vi "ActionOnStart.vi"(8 "error in (no error)":errorcluster, 11 "Channel Manager in":refnum<class "Channel Manager.lvclass">) -> (0 "error out":errorcluster, 3 "Channel Manager out":refnum<class "Channel Manager.lvclass">)   [LabVIEW 2024, in "Embedded TDMS Logger Engine.lvlib" / "Channel Manager.lvclass"]
uses:
  Channel Manager.lvclass
  Channel Manager.lvclass/Channel Manager.ctl
  Shared/File Classes/File/File.lvclass
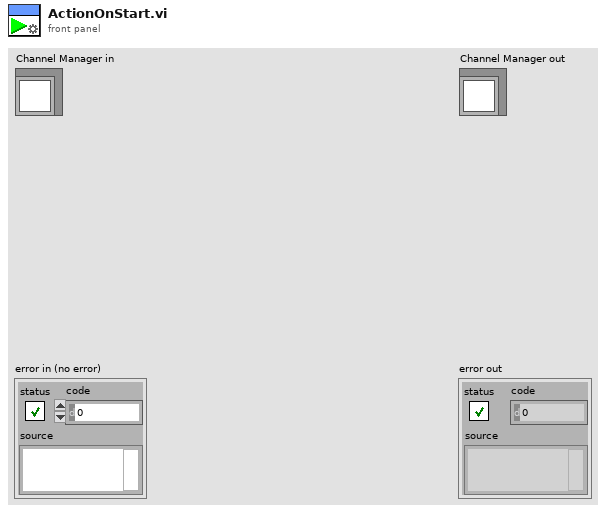
[diagram p1: front panel]
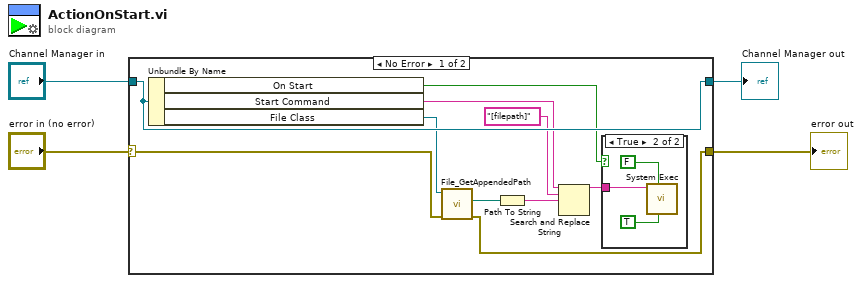
[diagram p0: block diagram]
diagram:
  n1 = case shown="No Error" "error in (no error)" {
    selector: "error in (no error)" -> [w11 w19]
    tunnel: [w10 w19] -> w3
    tunnel: [w14 w18] -> w1
    tunnel: "Channel Manager in" -> [w14 w18]
    frame No Error {
      n2 = Unbundle By Name(w14) -> ("On Start"=w13:bool, "Start Command"=w6:string, "File Class"=w12:refnum<class "File.lvclass">)
      n3 = call-dynamic "File_GetAppendedPath.vi"("error in (no error)"=w11, "File in"=w12) -> ("error out"=w10:errorcluster, "appended path"=w9:path)  [unwired: 7 in, 1 out]
      n4 = Path To String(path=w9) -> (string=w8:string)
      n5 = Search and Replace String(input string=w6, search string="[filepath]", replace string=w8) -> (result string=w7:string)  [unwired: 5 in, 3 out]
      n6 = case shown="True" w13 {
        tunnel: w7 -> [_ w15]
        frame False {
        }
        frame True {
          n7 = call <vilib>:"System Exec.vi"("run minimized? (F)"=TRUE, "wait until completion? (T)"=FALSE, "command line"=w15) -> ()  [unwired: 5 in, 4 out]
        }
      }
    }
    frame Error {
    }
  }
  "error out" <- w3
  "Channel Manager out" <- w1
